vi "多参数报警信息.vi"(8 "error in (no error)":errorcluster, 11 "data in":T1) -> (0 "error out":errorcluster)   [LabVIEW 2016, in "斯坦道多参数.lvlib"]
uses:
  <vilib>/Utility/sysdir.llb/System Directory Type.ctl
  <vilib>/addons/database/Auxilliary.llb/DB Tools Transaction.ctl
  <vilib>/addons/database/Auxilliary.llb/DB Tools Isolation Level.ctl
  <vilib>/addons/database/Connection.llb/DB Tools Open Connec (String).vi
  <vilib>/addons/database/Connection.llb/Conn Transaction.vi
  <vilib>/addons/database/NI_Database_API.lvlib
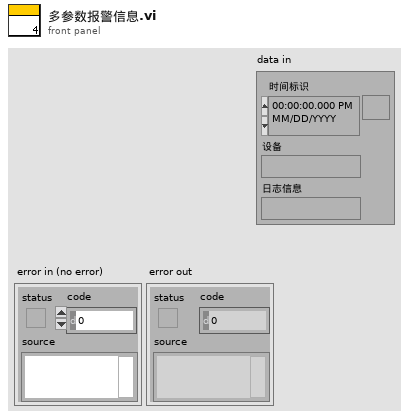
[diagram p1: front panel]
types:
  T1 = cluster{"时间标识":timestamp, "设备":string, "日志信息":string}
  T2 = typedef "NI_Database_API.lvlib/DB Tools Transaction.ctl" = enum16{"begin", "commit", "rollback"}
  T3 = typedef "NI_Database_API.lvlib/DB Tools Isolation Level.ctl" = enum16{"chaos", "read uncommitted", "read committed", "repeatable read", "serializable"}
  T4 = typedef "System Directory Type.ctl" = i32
  T5 = typedef "NI_Database_API.lvlib/Conn ObjectReference.ctl" = refnum<k1>
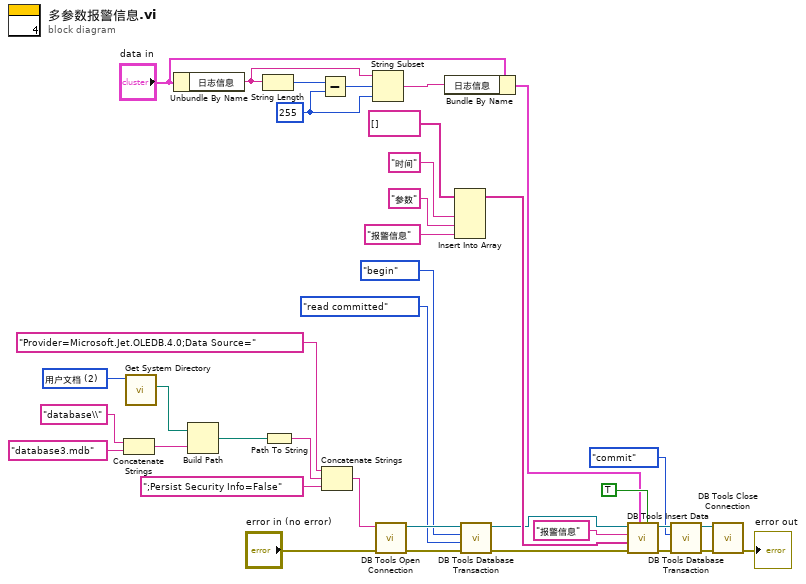
[diagram p0: block diagram]
diagram:
  w17 = 255 ("y")
  w36 = T4 2 items=["用户目录"=0, "用户桌面"=1, "用户文档"=2, "用户应用程序数据"=3, "用户设置"=4, "用户临时目录"=5, "公共文档"=6, "公共应用程序数据"=7, "公共设置"=8, "公共缓存"=13, "系统核心库"=9, "系统安装库"=10, "应用程序文件"=11, "启动盘根目录"=12] ("system directory type")
  n1 = Concatenate Strings("database\\" ("condition"), "database3.mdb" ("database")) -> (w28:string)
  n2 = call <vilib>:"Get System Directory.vi"("system directory type"=w36) -> ("system directory"=w34:path)  [unwired: 10 in]
  n3 = Unbundle By Name("data in") -> ("日志信息"=w16:string)
  n4 = Build Path(base path=w34, name or relative path=w28) -> (appended path=w33:path)
  n5 = String Length(string=w16) -> (length=w19:i32)
  n6 = Path To String(path=w33) -> (string=w32:string)
  n7 = Subtract(x=w19, y=w17) -> (x-y=w18:i32)
  n8 = Concatenate Strings("Provider=Microsoft.Jet.OLEDB.4.0;Data Source=" ("condition"), w32, ";Persist Security Info=False" ("condition")) -> (w30:string)
  n9 = String Subset(string=w16, offset (0)=w18, length (rest)=w17) -> (substring=w14:string)
  n10 = call-poly <vilib>:"DB Tools Open Connection.vi"("error in (no error)"="error in (no error)", "connection information"=w30) -> ("error out"=w11:errorcluster, "connection reference"=w27:T5)  [unwired: 6 in]
  n11 = Bundle By Name(cluster="data in", "日志信息"=w14) -> (w13:T1)
  n12 = Insert Into Array(array=string[] [], new element #1="时间", new element #2="参数" ("元素"), new element #3="报警信息") -> (w20:string[])  [unwired: 1 in]
  n13 = call-poly <vilib>:"DB Tools Database Transaction.vi"("error in (no error)"=w11, "isolation level (chaos)"=DB_Tools_Isolation_Level."read committed", "operation (begin)"=DB_Tools_Transaction."begin", "connection reference"=w27) -> ("error out"=w10:errorcluster, "connection reference out"=w12:T5)  [unwired: 2 in]
  n14 = call <vilib>:"DB Tools Insert Data.vi"("create table? (F)"=TRUE, "data"=w13, "error in (no error)"=w10, "columns"=w20, "table"="报警信息", "connection reference"=w12) -> ("error out"=w5:errorcluster, "connection reference out"=w7:T5)  [unwired: 4 in]
  n15 = call-poly <vilib>:"DB Tools Database Transaction.vi"("error in (no error)"=w5, "operation (begin)"=DB_Tools_Transaction."commit", "connection reference"=w7) -> ("error out"=w3:errorcluster, "connection reference out"=w6:T5)  [unwired: 3 in]
  n16 = call <vilib>:"DB Tools Close Connection.vi"("error in (no error)"=w3, "connection reference"=w6) -> ("error out"=→"error out":errorcluster)  [unwired: 5 in]
